vi "DSC Dashboard.vi"() -> ()   [LabVIEW 2016]
uses:
  <vilib>/addons/_JKI.lib/REST Client/classes/REST Client/HTTP Header.ctl
  OAuth/OO OAuth/scope_needed.ctl
  <vilib>/Platform/browser.llb/Open URL in Default Browser (string).vi
  <vilib>/regexp/Match Regular Expression.xnode
  <vilib>/addons/_JKI.lib/REST Client/classes/REST Client/REST Client.lvclass
  <vilib>/addons/_JKI.lib/Serialization/JSON/JKI JSON Serialization.lvlib
panel:
  out "Last Update":string
  in  "Go to Asana":bool
  in  "Add new value":bool
  in  "Update Button":bool
  in  "OK":bool
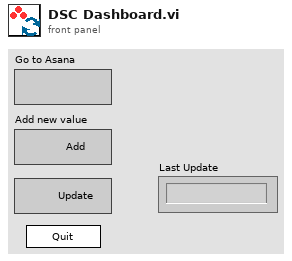
[diagram p1: front panel]
types:
  T1 = enum32{"Invalid", "Standard", "Closed", "Hidden", "Minimized", "Maximized"}
  T2 = enum32{"invalid app kind", "Development System", "Run Time System", "Student Edition", "Embedded LabVIEW", "Evaluation", "Custom"}
  T3 = cluster{"Client ID":string, "Client Secret":string, "Redirect URI":string, "Token Endpoint":string, "Scope":string}
  T4 = typedef "scope_needed.ctl" = enum16{"No", "Yes"}
  T5 = typedef "REST Client.lvlib/REST Client.lvclass/HTTP Header.ctl" = cluster{"header":string, "value":string}
  T6 = cluster{"Core":cluster{"Current VI Reference":refnum<vi>, "Close Panel on Exit?":bool}, "Access Token":string, "Auth Timeout":dbl, "Refresh Token":string, "DSC Data + GID":cluster{dbl, string}[], "headers":T5[]}
  T7 = cluster{"Current VI Reference":refnum<vi>, "Close Panel on Exit?":bool}
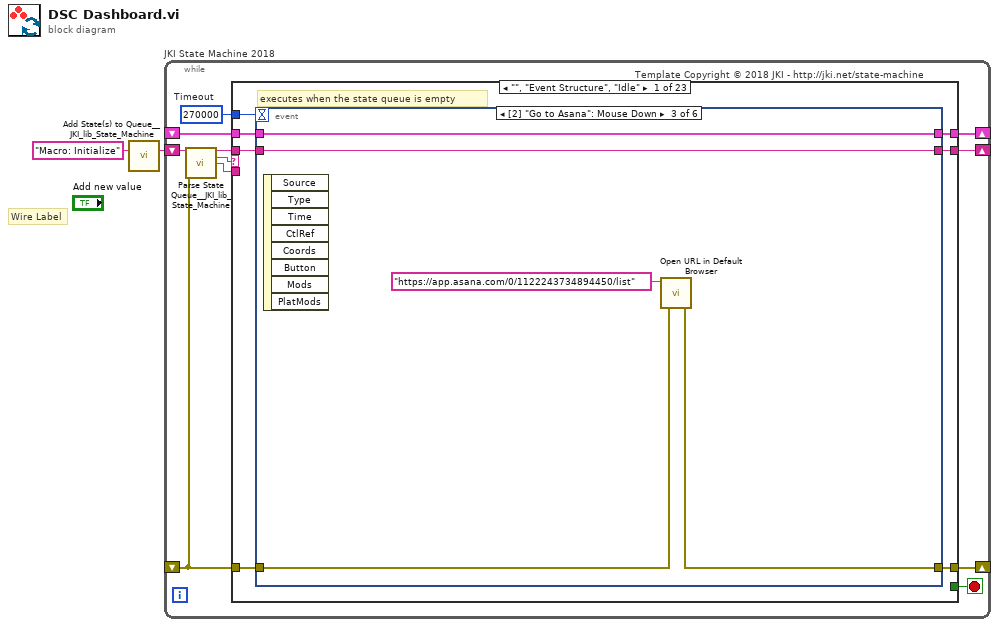
[diagram p0: block diagram]
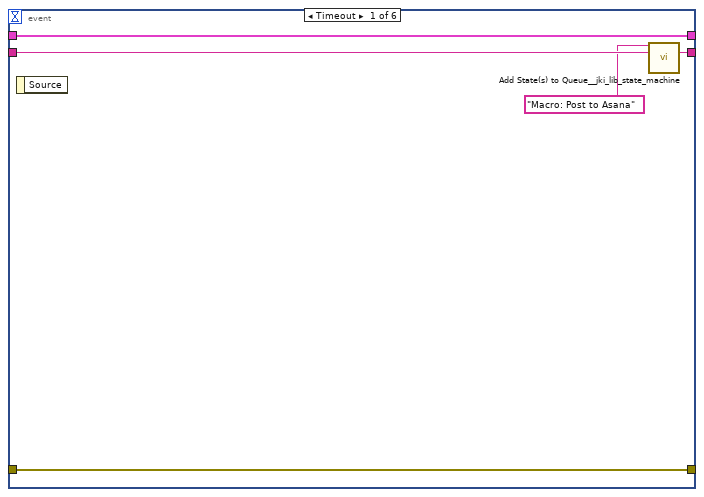
[diagram p2: hidden frame]
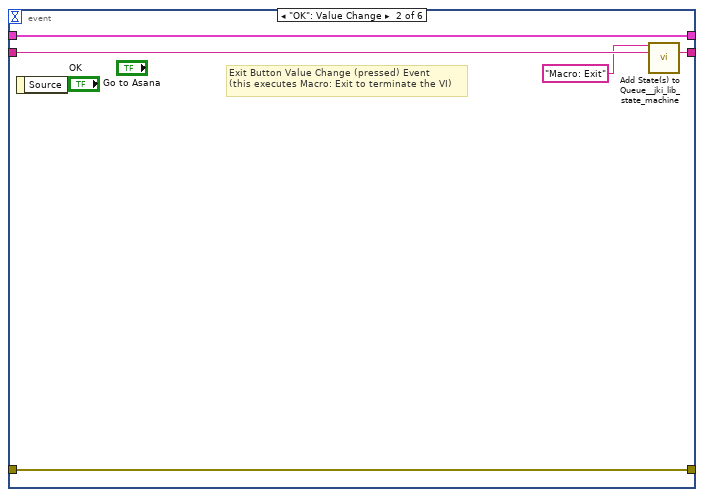
[diagram p3: hidden frame]
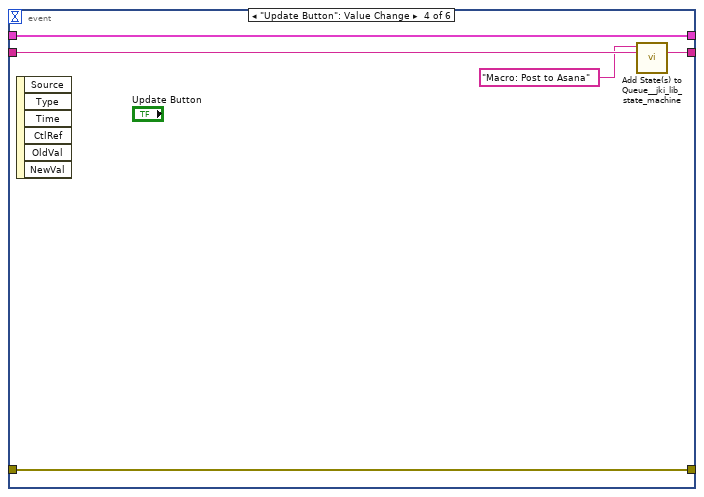
[diagram p4: hidden frame]
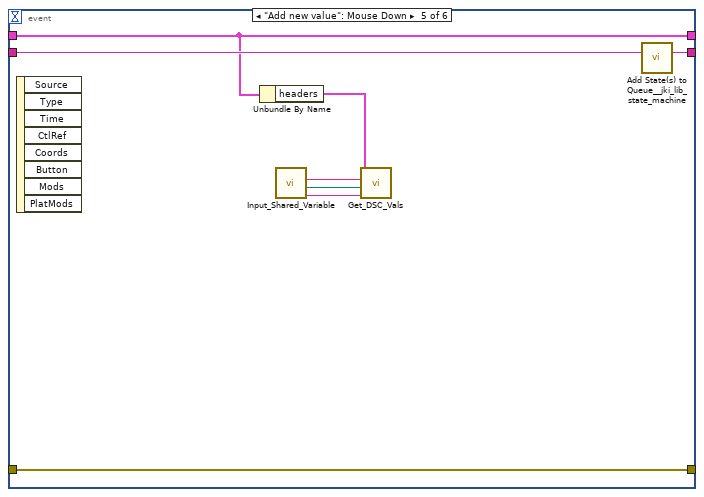
[diagram p5: hidden frame]
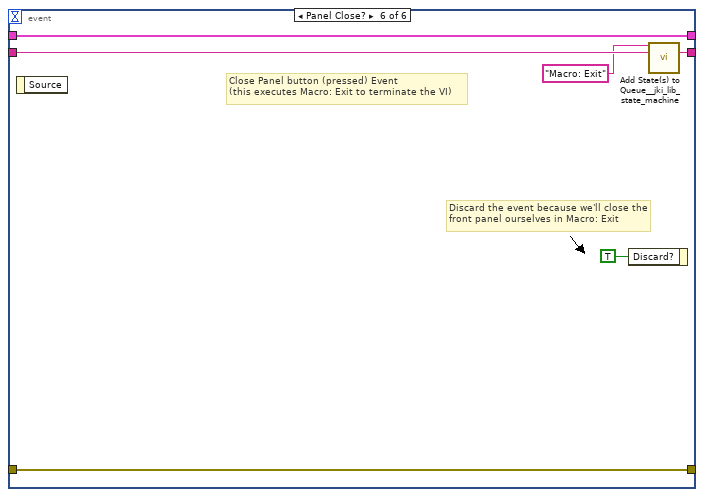
[diagram p6: hidden frame]
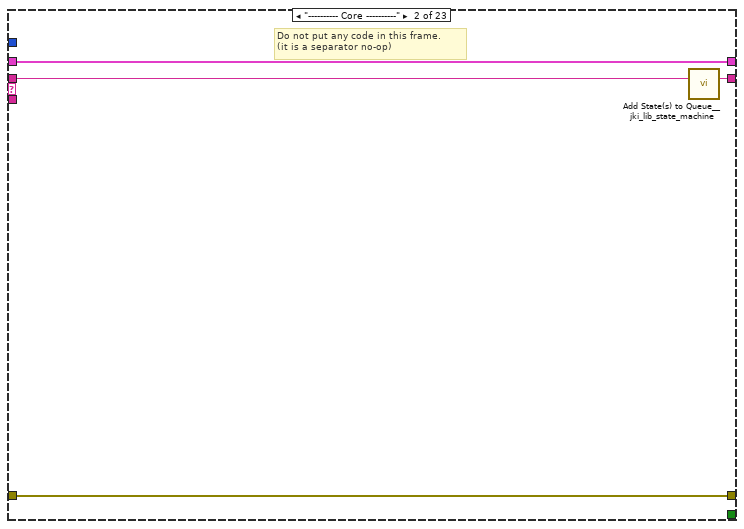
[diagram p7: hidden frame]
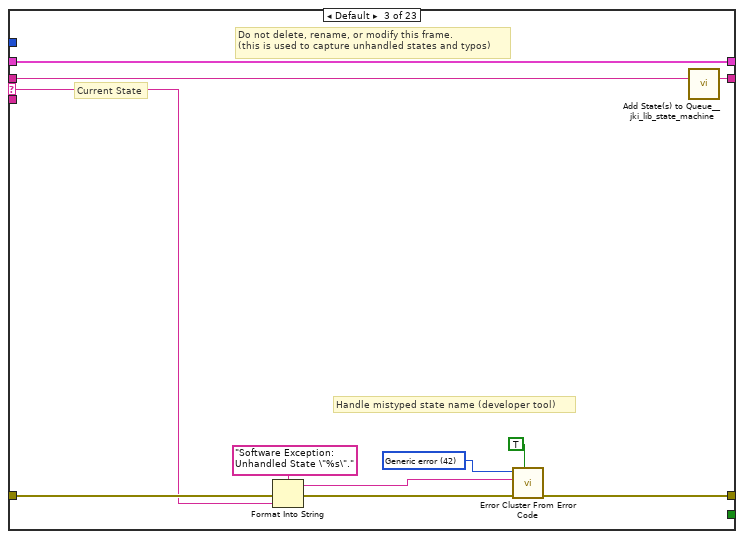
[diagram p8: hidden frame]
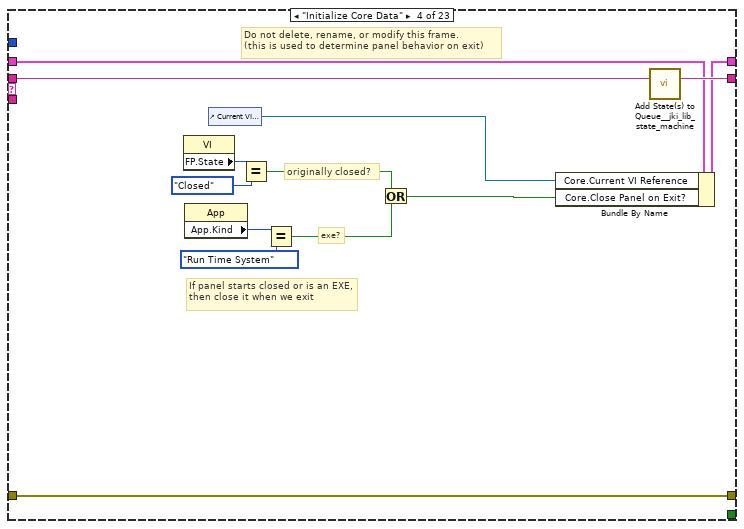
[diagram p9: hidden frame]
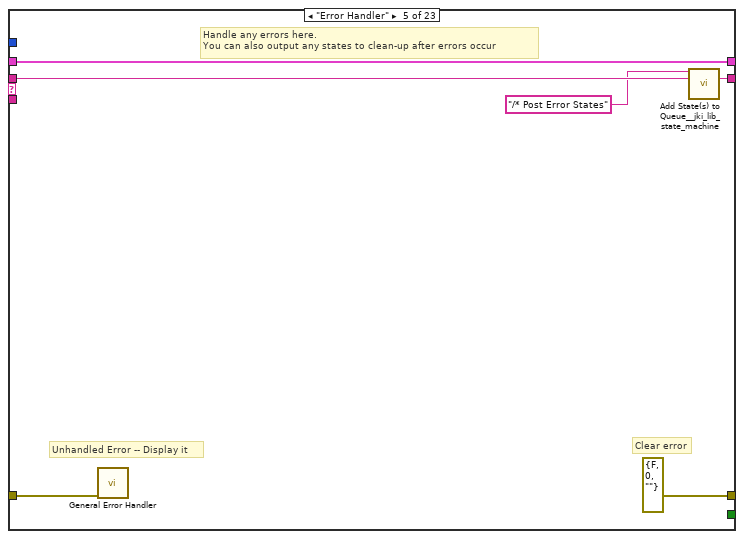
[diagram p10: hidden frame]
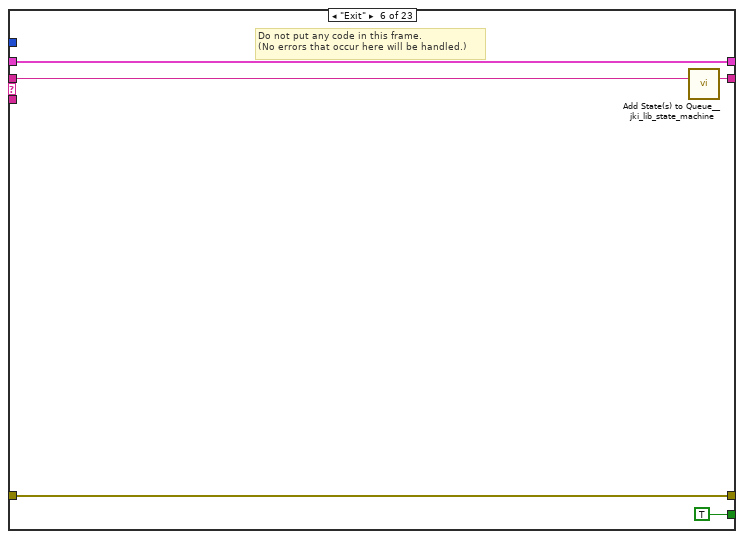
[diagram p11: hidden frame]
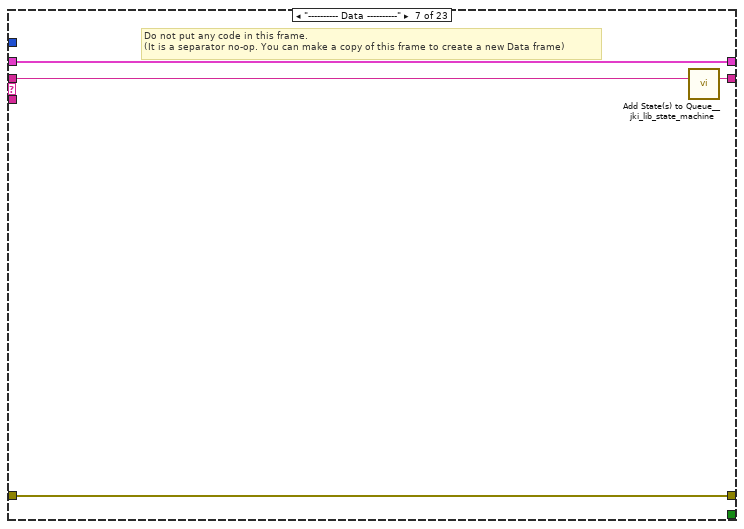
[diagram p12: hidden frame]
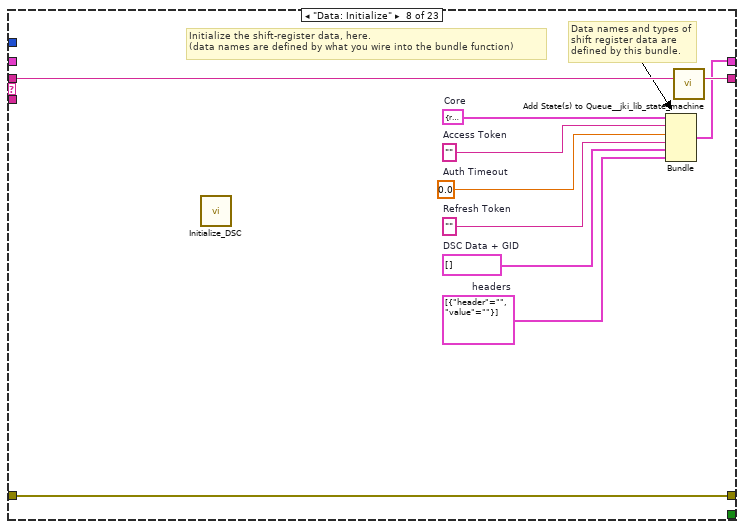
[diagram p13: hidden frame]
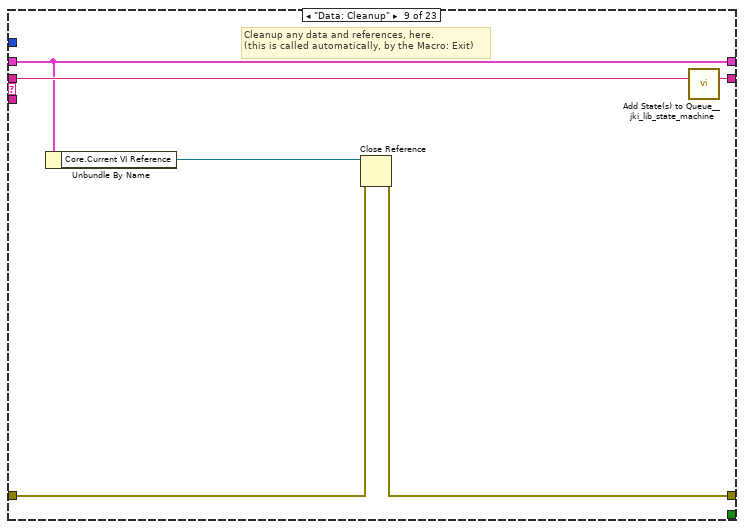
[diagram p14: hidden frame]
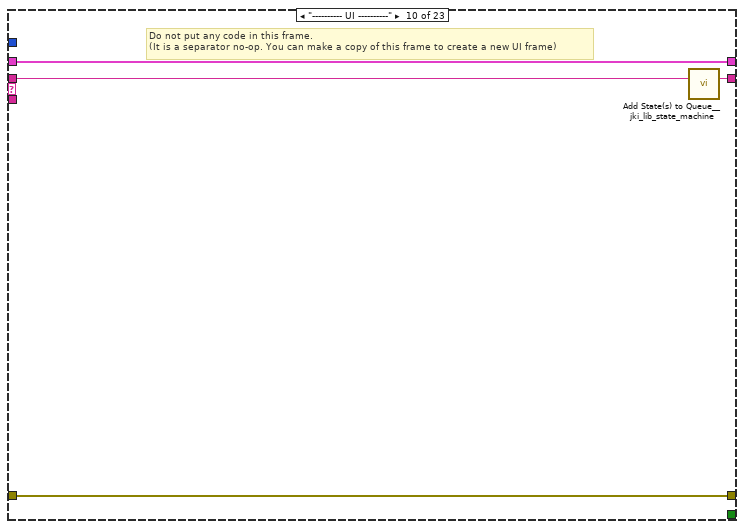
[diagram p15: hidden frame]
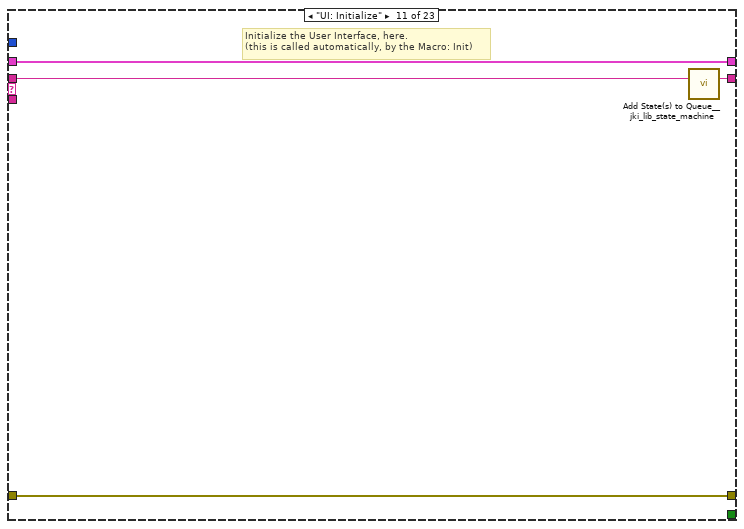
[diagram p16: hidden frame]
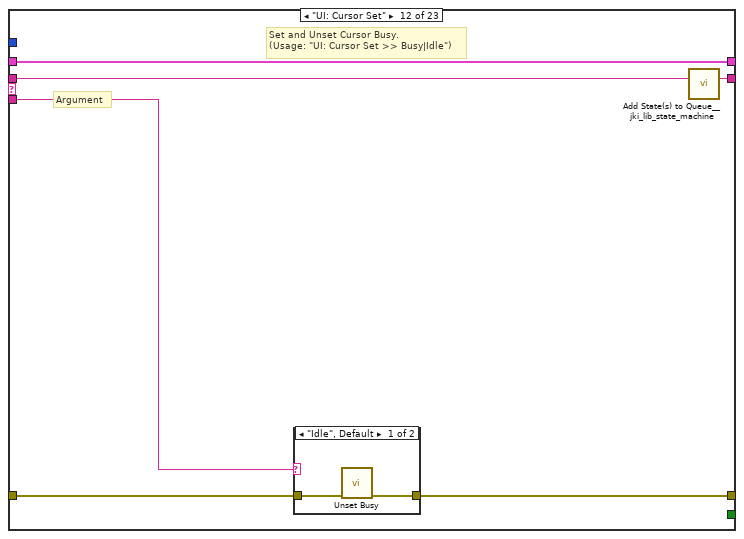
[diagram p17: hidden frame]
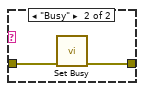
[diagram p18: hidden frame]
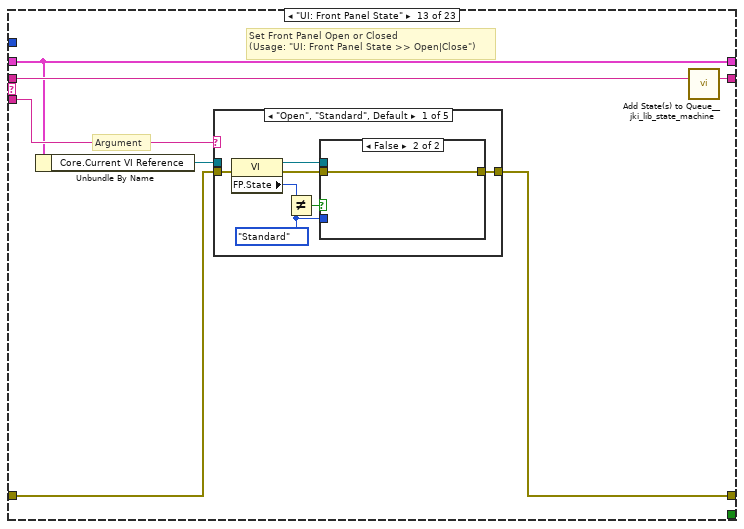
[diagram p19: hidden frame]
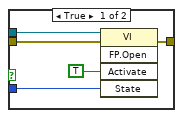
[diagram p20: hidden frame]
diagram:
  # "Wire Label"
  n1 = call <vilib>:"Add State(s) to Queue__JKI_lib_State_Machine.vi"("State(s) in (\"\")"="Macro: Initialize") -> ("States Out"=w2:string)  [unwired: 14 in]
  n2 = while "JKI State Machine 2018" {
    shift-right: [w3] -> _
    shift-left: _ -> [w6]
    shift-right: [w9] -> _
    shift-left: _ -> [w4]
    shift-right: [w8] -> _
    shift-left: w2 -> [w10]
    stop <- w7 stop-if-true
    w5 = 270000  # Timeout
    # "Template Copyright © 2018 JKI - http://jki.net/state-machine"
    n3 = call <vilib>:"Parse State Queue__JKI_lib_State_Machine.vi"("State Queue"=w10, "Error In (no error)"=w4) -> ("Remaining States"=w12:string, "Current State"=w13:string, "Arguments"=w11:string)  [unwired: 11 in]
    n4 = case shown="\"\", \"Event Structure\", \"Idle\"" w13 {
      selector: w13 -> [_ _ w59 _ _ _ _ _ _ _ _ _ _ _ _ _ _ _ _ _ _ _ _]
      tunnel: w12 -> [w20 w58 w63 w82 w88 w93 w97 w107 w113 w117 w121 w127 w138 w202 w207 w212 w222 w226 w237 w253 w269 w287 w297]
      tunnel: w11 -> [_ _ _ _ _ _ _ _ _ _ _ w122 w133 _ _ _ _ _ _ _ _ _ _]
      tunnel: w6 -> [w18 w55 w61 w71 w85 w91 w94 _ w109 w114 w119 w125 w132 w199 w204 w209 w214 w223 w228 w250 w255 w284 w294]
      tunnel: [w17 w56 w65 w80 errorcluster {"status"=FALSE, "code"=0, "source"=""} ("error out") w90 w95 w105 w110 w115 w118 w123 w135 w200 w205 w210 w220 w224 w231 w251 w260 w285 w295] -> w9
      tunnel: w4 -> [w16 w56 w64 w80 w84 w90 w95 w105 w111 w115 w118 w124 w136 w200 w205 w210 w220 w224 w232 w251 w265 w285 w295]
      tunnel: [w19 w57 w62 w81 w87 w92 w96 w106 w112 w116 w120 w126 w137 w201 w206 w211 w221 w225 w236 w252 w268 w286 w296] -> w8
      tunnel: [_ _ _ _ _ TRUE _ _ _ _ _ _ _ _ _ _ _ _ _ _ _ _ _] -> w7
      tunnel: w5 -> [w14 _ _ _ _ _ _ _ _ _ _ _ _ _ _ _ _ _ _ _ _ _ _]
      tunnel: [w15 w55 w61 w70 w85 w91 w94 w98 w109 w114 w119 w125 w132 w199 w204 w209 w214 w223 w227 w250 w254 w284 w294] -> w3
      frame "", "Event Structure", "Idle" {
        # "executes when the state queue is empty"
        n5 = event shown="[2] \"Go to Asana\": Mouse Down" {
          selector: _ -> [_ _ _ _ _ _]
          dyn-events: _ -> [_ _ _ _ _ _]
          timeout: w14 -> [_ _ _ _ _ _]
          tunnel: w20 -> [w25 w30 w34 w38 w47 w54]
          tunnel: [w24 w29 w34 w39 w48 w53] -> w19
          tunnel: w18 -> [w22 w27 w35 w40 w44 w51]
          tunnel: [w23 w28 w31 w36 w46 w52] -> w17
          tunnel: w16 -> [w23 w28 w32 w36 w46 w52]
          tunnel: [w22 w27 w35 w40 w44 w51] -> w15
          event Timeout {
            n6 = event-data() -> ()  [unwired: 1 in, 1 out]
            n7 = call <vilib>:"Add State(s) to Queue__jki_lib_state_machine.vi"("State(s) in Front (\"\")"="Macro: Post to Asana" ("State(s) in Front (\"\")"), "State(s) in (\"\")"=w25) -> ("States Out"=w24:string)  [unwired: 13 in]
          }
          event "OK": Value Change {
            # "Exit Button Value Change (pressed) Event\n(this executes Macro: Exit to terminate the VI)"
            n8 = event-data() -> ()  [unwired: 1 in, 1 out]
            n9 = call <vilib>:"Add State(s) to Queue__jki_lib_state_machine.vi"("State(s) in Front (\"\")"="Macro: Exit", "State(s) in (\"\")"=w30) -> ("States Out"=w29:string)  [unwired: 13 in]
          }
          event "Go to Asana": Mouse Down {
            n10 = event-data() -> ()  [unwired: 1 in, 8 out]
            n11 = call-poly <vilib>:"Open URL in Default Browser.vi"("error in (no error)"=w32, "URL"="https://app.asana.com/0/1122243734894450/list") -> ("error out"=w31:errorcluster)  [unwired: 4 in, 1 out]
          }
          event "Update Button": Value Change {
            n12 = event-data() -> ()  [unwired: 1 in, 6 out]
            n13 = call <vilib>:"Add State(s) to Queue__jki_lib_state_machine.vi"("State(s) in Front (\"\")"="Macro: Post to Asana", "State(s) in (\"\")"=w38) -> ("States Out"=w39:string)  [unwired: 13 in]
          }
          event "Add new value": Mouse Down {
            n14 = event-data() -> ()  [unwired: 1 in, 8 out]
            n15 = Unbundle By Name(w44) -> ("headers"=w45:T5[])
            n16 = call "Input_Shared_Variable.vi"() -> ("Machine Out"=w41:string, "Shared Variable Out"=w42:refnum<k21>, "Type out"=w43:string)  [unwired: 9 in]
            n17 = call "Get_DSC_Vals.vi"("Machine"=w41, "Shared Variable Control"=w42, "Name"=w43, "Authorization Header"=w45) -> ()  [unwired: 8 in]
            n18 = call <vilib>:"Add State(s) to Queue__jki_lib_state_machine.vi"("State(s) in (\"\")"=w47) -> ("States Out"=w48:string)  [unwired: 14 in]
          }
          event Panel Close? {
            # "Discard the event because we'll close the front panel ourselves in Macro: Exit"
            # "Close Panel button (pressed) Event\n(this executes Macro: Exit to terminate the VI)"
            n19 = event-data() -> ()  [unwired: 1 in, 1 out]
            n20 = event-data("Discard?"=TRUE) -> ()  [unwired: 1 in, 1 out]
            n21 = call <vilib>:"Add State(s) to Queue__jki_lib_state_machine.vi"("State(s) in Front (\"\")"="Macro: Exit", "State(s) in (\"\")"=w54) -> ("States Out"=w53:string)  [unwired: 13 in]
          }
        }
      }
      frame "---------- Core ----------" {
        # "Do not put any code in this frame.\n(it is a separator no-op)"
        n22 = call <vilib>:"Add State(s) to Queue__jki_lib_state_machine.vi"("State(s) in (\"\")"=w58) -> ("States Out"=w57:string)  [unwired: 14 in]
      }
      frame Default {
        w68 = 42 items=["No error", "Argument error", "Memory is full", "Out of zone", "End of file", "File already open", "Generic file I/O error", "File not found", "File permission error", "Disk is full", "Duplicate path", "Too many files open", "System feature not enabled", "Resource file not found", "Cannot add resource", "Resource not found", "Image not found", "Image memory error", "Pen does not exist", "Config type invalid", "Config token not found", "Config parse error", "Config memory error", "Bad external code format", "Bad external code offset", "External code not present", "Null window", "Destroy window error", "Null menu", "Print aborted", "Bad print record", "Print driver error", "Windows error during printing", "Memory error during printing", "Print dialog error", "Generic print error", "Invalid device refnum", "Device not found", "Device parameter error", "Device unit error", "Cannot open device", "Device call aborted", "Generic error", "Cancelled by user", "Object ID too low", "Object ID too high", "Object not in heap", "Unknown heap", "Unknown object (invalid DefProc)", "Unknown object (DefProc not in table)", "Message out of range", "Invalid (null) method", "Unknown message", "Manager call not supported", "Bad address", "Network operation in progress", "Network operation timed out", "Connection is busy", "Network attribute not supported", "Network error", "Address in use", "System out of memory", "Connection aborted", "Connection refused", "Not connected", "Already connected", "Connection closed", "Initialization error (interapplication manager)", "Bad occurrence", "Wait on unbound occurrence handler", "Occurrence queue overflow", "Datalog type conflict", "Unused", "Unrecognized type (interapplication manager)", "Memory corrupt", "Failed to make temporary DLL", "Old CIN version", "Drag socket not found", "Failed to load drop-object", "Failed to register OLE object", "Failed to release OLE object", "Format specifier type mismatch", "Unknown format specifier", "Too few format specifiers", "Too many format specifiers", "Scan failed", "Newer CIN version", "Error converting to variant", "Runtime menu error", "Password tampered", "Variant attribute not found", "Incompatible variant data type", "Event data is not available", "Event Store is not present", "Occurrence is not found", "Event Queue is not created", "Event info is not available", "Refnum passed is NULL", "Error retrieving Class GUID", "Error retrieving CoClass GUID", "Error retrieving TypeLib GUID.", "Bad built application magic bytes.", "Specific driver is different from the specific driver associated with the Logical Name.", "There is no session opened to the class driver.", "Max Error", "MAX - Error with config objects", "MAX - Error loading configuration", "MAX - Group not supported"]
        # "Current State"
        # "Do not delete, rename, or modify this frame.\n(this is used to capture unhandled states and typos)"
        # "Handle mistyped state name (developer tool)"
        n23 = Format Into String(format string="Software Exception: Unhandled State \"%s\"." ("message"), error in=w64, w59) -> (resulting string=w67:string, error out=w66:errorcluster)  [unwired: 1 in]
        n24 = call <vilib>:"Error Cluster From Error Code.vi"("show call chain? (False)"=TRUE, "error in (no error)"=w66, "error message (\"\")"=w67, "error code (0)"=w68) -> ("error out"=w65:errorcluster)  [unwired: 5 in]
        n25 = call <vilib>:"Add State(s) to Queue__jki_lib_state_machine.vi"("State(s) in (\"\")"=w63) -> ("States Out"=w62:string)  [unwired: 14 in]
      }
      frame "Initialize Core Data" {
        # "Do not delete, rename, or modify this frame.\n(this is used to determine panel behavior on exit)"
        # "originally closed?"
        # "exe?"
        # "If panel starts closed or is an EXE, then close it when we exit"
        n26 = property class="VI"() -> ("FP.State"=w74:T1)  [unwired: 2 in, 2 out]
        n27 = property class="App"() -> ("App.Kind"=w79:T2)  [unwired: 2 in, 2 out]
        n28 = control-ref of="Current VI Reference"() -> (w75:refnum<vi>)
        n29 = Equal?(x=w74, y=T1."Closed" ("Front Panel Window:State")) -> (x = y?=w72:bool)
        n30 = Equal?(x=w79, y=T2."Run Time System" ("Application:Kind")) -> (x = y?=w77:bool)
        n31 = Or(x=w72, y=w77) -> (x .or. y?=w76:bool)
        n32 = Bundle By Name(cluster=w71, "Core.Current VI Reference"=w75, "Core.Close Panel on Exit?"=w76) -> (w70:T6)
        n33 = call <vilib>:"Add State(s) to Queue__jki_lib_state_machine.vi"("State(s) in (\"\")"=w82) -> ("States Out"=w81:string)  [unwired: 14 in]
      }
      frame "Error Handler" {
        # "Unhandled Error -- Display it"
        # "Handle any errors here.\nYou can also output any states to clean-up after errors occur"
        # "Clear error"
        n34 = call <vilib>:"General Error Handler.vi"("error in (no error)"=w84) -> ()  [unwired: 10 in, 5 out]
        n35 = call <vilib>:"Add State(s) to Queue__jki_lib_state_machine.vi"("State(s) in Front (\"\")"="/* Post Error States", "State(s) in (\"\")"=w88) -> ("States Out"=w87:string)  [unwired: 13 in]
      }
      frame "Exit" {
        # "Do not put any code in this frame.\n(No errors that occur here will be handled.)"
        n36 = call <vilib>:"Add State(s) to Queue__jki_lib_state_machine.vi"("State(s) in (\"\")"=w93) -> ("States Out"=w92:string)  [unwired: 14 in]
      }
      frame "---------- Data ----------" {
        # "Do not put any code in this frame.\n(It is a separator no-op. You can make a copy of this frame to create a new Data frame)"
        n37 = call <vilib>:"Add State(s) to Queue__jki_lib_state_machine.vi"("State(s) in (\"\")"=w97) -> ("States Out"=w96:string)  [unwired: 14 in]
      }
      frame "Data: Initialize" {
        w99 = cluster{dbl, string}[] []  # DSC Data + GID
        w100 = T5[] [{"header"="", "value"=""}]  # headers
        w101 = ""  # Refresh Token
        w102 = ""  # Access Token
        w103 = 0.0  # Auth Timeout
        w104 = T7 {"Current VI Reference"=refnum, "Close Panel on Exit?"=FALSE}  # Core
        # "Data names and types of shift register data are defined by this bundle."
        # "Initialize the shift-register data, here.\n(data names are defined by what you wire into the bundle function)"
        n38 = call "Initialize_DSC.vi"() -> ()  [unwired: 12 in]
        n39 = Bundle("Core"=w104, "Access Token"=w102, "Auth Timeout"=w103, "Refresh Token"=w101, "DSC Data + GID"=w99, "headers"=w100) -> (w98:T6)  [unwired: 1 in]
        n40 = call <vilib>:"Add State(s) to Queue__jki_lib_state_machine.vi"("State(s) in (\"\")"=w107) -> ("States Out"=w106:string)  [unwired: 14 in]
      }
      frame "Data: Cleanup" {
        # "Cleanup any data and references, here.\n(this is called automatically, by the Macro: Exit)"
        n41 = Unbundle By Name(w109) -> ("Core.Current VI Reference"=w108:refnum<vi>)
        n42 = Close Reference(reference=w108, error in (no error)=w111) -> (error out=w110:errorcluster)
        n43 = call <vilib>:"Add State(s) to Queue__jki_lib_state_machine.vi"("State(s) in (\"\")"=w113) -> ("States Out"=w112:string)  [unwired: 14 in]
      }
      frame "---------- UI ----------" {
        # "Do not put any code in this frame.\n(It is a separator no-op. You can make a copy of this frame to create a new UI frame)"
        n44 = call <vilib>:"Add State(s) to Queue__jki_lib_state_machine.vi"("State(s) in (\"\")"=w117) -> ("States Out"=w116:string)  [unwired: 14 in]
      }
      frame "UI: Initialize" {
        # "Initialize the User Interface, here.\n(this is called automatically, by the Macro: Init)"
        n45 = call <vilib>:"Add State(s) to Queue__jki_lib_state_machine.vi"("State(s) in (\"\")"=w121) -> ("States Out"=w120:string)  [unwired: 14 in]
      }
      frame "UI: Cursor Set" {
        # "Argument"
        # "Set and Unset Cursor Busy.\n(Usage: \"UI: Cursor Set >> Busy|Idle\")"
        n46 = case shown="\"Idle\", Default" w122 {
          tunnel: w124 -> [w129 w131]
          tunnel: [w128 w130] -> w123
          frame "Idle", Default {
            n47 = call <vilib>:"Unset Busy.vi"("error in (no error)"=w129) -> ("error out"=w128:errorcluster)  [unwired: 10 in]
          }
          frame "Busy" {
            n48 = call <vilib>:"Set Busy.vi"("error in (no error)"=w131) -> ("error out"=w130:errorcluster)  [unwired: 9 in, 1 out]
          }
        }
        n49 = call <vilib>:"Add State(s) to Queue__jki_lib_state_machine.vi"("State(s) in (\"\")"=w127) -> ("States Out"=w126:string)  [unwired: 14 in]
      }
      frame "UI: Front Panel State" {
        # "Argument"
        # "Set Front Panel Open or Closed\n(Usage: \"UI: Front Panel State >> Open|Close\")"
        n50 = Unbundle By Name(w132) -> ("Core.Current VI Reference"=w134:refnum<vi>)
        n51 = case shown="\"Open\", \"Standard\", Default" w133 {
          tunnel: w136 -> [w144 w157 w168 w180 w192]
          tunnel: [w145 w158 w169 w181 w193] -> w135
          tunnel: w134 -> [_ _ _ _ _]
          frame "Open", "Standard", Default {
            w139 = T1."Standard" ("State")
            n52 = property class="VI"(error in=w144) -> (reference out=w142:refnum<vi>, error out=w143:errorcluster, "FP.State"=w141:T1)  [unwired: 1 in]
            n53 = Not Equal?(x=w141, y=w139) -> (x != y?=w140:bool)
            n54 = case shown="False" w140 {
              tunnel: [w149 w151] -> w145
              tunnel: w143 -> [w148 w151]
              tunnel: w142 -> [w147 _]
              tunnel: w139 -> [w146 _]
              frame True {
                n55 = invoke class="VI" method="FP.Open"(reference=w147, error in=w148, "Activate"=TRUE, "State"=w146) -> (error out=w149:errorcluster)  [unwired: 1 in, 4 out]
              }
              frame False {
              }
            }
          }
          frame "Close", "Closed" {
            n56 = property class="VI"(error in=w157) -> (reference out=w155:refnum<vi>, error out=w156:errorcluster, "FP.State"=w153:T1)  [unwired: 1 in]
            n57 = Not Equal?(x=w153, y=T1."Closed" ("Front Panel Window:State")) -> (x != y?=w152:bool)
            n58 = case shown="True" w152 {
              tunnel: [w159 w162] -> w158
              tunnel: w156 -> [w159 w161]
              tunnel: w155 -> [_ w160]
              frame False {
              }
              frame True {
                n59 = invoke class="VI" method="FP.Close"(reference=w160, error in=w161) -> (error out=w162:errorcluster)  [unwired: 1 in, 2 out]
              }
            }
          }
          frame "Hidden", "Hide" {
            w163 = T1."Hidden" ("State")
            n60 = property class="VI"(error in=w168) -> (reference out=w166:refnum<vi>, error out=w167:errorcluster, "FP.State"=w165:T1)  [unwired: 1 in]
            n61 = Not Equal?(x=w165, y=w163) -> (x != y?=w164:bool)
            n62 = case shown="True" w164 {
              tunnel: [w173 w174] -> w169
              tunnel: w167 -> [w172 w174]
              tunnel: w166 -> [w171 _]
              tunnel: w163 -> [w170 _]
              frame True {
                n63 = invoke class="VI" method="FP.Open"(reference=w171, error in=w172, "State"=w170) -> (error out=w173:errorcluster)  [unwired: 2 in, 4 out]
              }
              frame False {
              }
            }
          }
          frame "Minimize", "Minimized" {
            w175 = T1."Minimized" ("State")
            n64 = property class="VI"(error in=w180) -> (reference out=w178:refnum<vi>, error out=w179:errorcluster, "FP.State"=w177:T1)  [unwired: 1 in]
            n65 = Not Equal?(x=w177, y=w175) -> (x != y?=w176:bool)
            n66 = case shown="True" w176 {
              tunnel: [w185 w186] -> w181
              tunnel: w179 -> [w184 w186]
              tunnel: w178 -> [w183 _]
              tunnel: w175 -> [w182 _]
              frame True {
                n67 = invoke class="VI" method="FP.Open"(reference=w183, error in=w184, "State"=w182) -> (error out=w185:errorcluster)  [unwired: 2 in, 4 out]
              }
              frame False {
              }
            }
          }
          frame "Maximize", "Maximized" {
            w187 = T1."Maximized" ("State")
            n68 = property class="VI"(error in=w192) -> (reference out=w190:refnum<vi>, error out=w191:errorcluster, "FP.State"=w189:T1)  [unwired: 1 in]
            n69 = Not Equal?(x=w189, y=w187) -> (x != y?=w188:bool)
            n70 = case shown="True" w188 {
              tunnel: [w197 w198] -> w193
              tunnel: w191 -> [w196 w198]
              tunnel: w190 -> [w195 _]
              tunnel: w187 -> [w194 _]
              frame True {
                n71 = invoke class="VI" method="FP.Open"(reference=w195, error in=w196, "State"=w194) -> (error out=w197:errorcluster)  [unwired: 2 in, 4 out]
              }
              frame False {
              }
            }
          }
        }
        n72 = call <vilib>:"Add State(s) to Queue__jki_lib_state_machine.vi"("State(s) in (\"\")"=w138) -> ("States Out"=w137:string)  [unwired: 14 in]
      }
      frame "---------- Macro ----------" {
        # "Do not put any code in this frame.\n(It is a separator no-op. You can make a copy of this frame to create a new Macro frame)"
        n73 = call <vilib>:"Add State(s) to Queue__jki_lib_state_machine.vi"("State(s) in (\"\")"=w202) -> ("States Out"=w201:string)  [unwired: 14 in]
      }
      frame "Macro: Post to Asana" {
        # "Do not put any code in this frame.\n(It is a separator no-op. You can make a copy of this frame to create a new Macro frame)"
        n74 = call <vilib>:"Add State(s) to Queue__jki_lib_state_machine.vi"("State(s) in Front (\"\")"="Authorization: Handle\nDSC: Get DSC Values\nAsana: Post Values" ("State(s) in Front (\"\")"), "State(s) in (\"\")"=w207) -> ("States Out"=w206:string)  [unwired: 13 in]
      }
      frame "Macro: Initialize" {
        w208 = "Data: Initialize\nInitialize Core Data\nUI: Initialize\nUI: Front Panel State >> Open\nMacro: Post to Asana"  # Data: Initialize Initialize Core Data UI: Initialize UI: Front Panel State >> Open Macro: Post to Asana
        # "Initialization Macro\n(This is called once, when the VI starts)"
        n75 = call <vilib>:"Add State(s) to Queue__jki_lib_state_machine.vi"("State(s) in Front (\"\")"=w208, "State(s) in (\"\")"=w212) -> ("States Out"=w211:string)  [unwired: 13 in]
      }
      frame "Macro: Exit" {
        # "Exit Macro\n(This is called once, when the VI exits)"
        n76 = Unbundle By Name(w214) -> ("Core.Close Panel on Exit?"=w213:bool)
        n77 = Select(t="UI: Front Panel State >> Close", s=w213, f="") -> (s? t:f=w217:string)
        n78 = call <vilib>:"Add State(s) to Queue__jki_lib_state_machine.vi"("State(s) in (\"\")"=w217, "State(s) at Back (\"\")"="Data: Cleanup\nExit") -> ("States Out"=w215:string)  [unwired: 13 in]
        n79 = call <vilib>:"Add State(s) to Queue__jki_lib_state_machine.vi"("State(s) in Front (\"\")"=w215, "State(s) in (\"\")"=w222) -> ("States Out"=w221:string)  [unwired: 13 in]
      }
      frame "---------- Authorization ----------" {
        # "Template Separator\n(You can make a copy of, or modify, this frame)"
        n80 = call <vilib>:"Add State(s) to Queue__jki_lib_state_machine.vi"("State(s) in (\"\")"=w226) -> ("States Out"=w225:string)  [unwired: 14 in]
      }
      frame "Authorization: Handle" {
        # "If it is, reauthenticate.\nIf not, do nothing."
        # "Check if the current time is\ngreater than the authentication\ndeadline"
        n81 = Get Date/Time In Seconds() -> (seconds since 1Jan1904=w235:timestamp)
        n82 = Unbundle By Name(w228) -> ("Auth Timeout"=w229:dbl, "Refresh Token"=w230:string)
        n83 = To Double Precision Float(number=w235) -> (double precision float=w233:dbl)
        n84 = Less Or Equal?(x=w229, y=w233) -> (x <= y?=w234:bool)
        n85 = case shown="True" w234 {
          tunnel: w232 -> [w239 w248]
          tunnel: [w239 w247] -> w231
          tunnel: [w238 w246] -> w227
          tunnel: w230 -> [_ _]
          tunnel: w228 -> [w238 w242]
          frame False {
          }
          frame True {
            n86 = call "Authenticate.vi"("error in (no error)"=w248, "Authentication Info"=T3 {"Client ID"="1108428692000476", "Client Secret"="803bdca1138fccb00921b8f346728904", "Redirect URI"="https://app.asana.com/api/1.0", "Token Endpoint"="https://app.asana.com/-/oauth_token", "Scope"=""}, "Scope Needed?"=scope_needed."No") -> ("error out"=w247:errorcluster, "Refresh Token"=w243:string, "Timeout"=w249:dbl, "Access Token"=w240:string)  [unwired: 5 in]
            n87 = call "Authentication_Header_Handler.vi"("String"=w240) -> ("output array"=w241:T5[])  [unwired: 10 in]
            n88 = Bundle By Name(cluster=w242, "headers"=w241, "Auth Timeout"=w249, "Refresh Token"=w243) -> (w246:T6)
          }
        }
        n89 = call <vilib>:"Add State(s) to Queue__jki_lib_state_machine.vi"("State(s) in (\"\")"=w237) -> ("States Out"=w236:string)  [unwired: 14 in]
      }
      frame "---------- DSC ----------" {
        # "Template Separator\n(You can make a copy of, or modify, this frame)"
        n90 = call <vilib>:"Add State(s) to Queue__jki_lib_state_machine.vi"("State(s) in (\"\")"=w253) -> ("States Out"=w252:string)  [unwired: 14 in]
      }
      frame "DSC: Get DSC Values" {
        w258 = cluster{string, string}[] []
        n91 = call <vilib>:"Application Directory.vi"() -> ("Application Directory"=w264:path)
        n92 = Build Path(base path=w264, name or relative path="DSC_Variables.json") -> (appended path=w267:path)
        n93 = Read from Text File(file (use dialog)=w267, error in=w265) -> (text=w259:string, error out=w262:errorcluster)  [unwired: 2 in, 2 out]
        n94 = call <vilib>:"Unflatten From JSON String.vi"("Type and Defaults"=w258, "error in (no error)"=w262, "JSON String"=w259) -> ("error out"=w261:errorcluster, "Variant"=w263:variant)  [unwired: 7 in]
        n95 = Variant To Data(error in=w261, type=w258, Variant=w263) -> (data=w256:cluster{string, string}[], error out=w260:errorcluster)
        n96 = for {
          tunnel: [w278] -> w257 mode=indexing
          tunnel: w256 -> [w276] mode=indexing
          n97 = Unbundle(w276) -> (w275:string, w274:string)
          n98 = Variant To Data(type=refnum<k21> refnum ("shared variable refnum in"), Variant=w275) -> (data=w282:refnum<k21>)  [unwired: 1 in, 1 out]
          n99 = shared-variable-open(w282, 0.0) -> (w281:refnum<k21>, w273:errorcluster)  [unwired: 2 in]
          n100 = shared-variable-read(w281) -> (w280:refnum<k21>, w272:errorcluster, w279:dbl)  [unwired: 1 in, 1 out]
          n101 = call <vilib>:"Clear Errors.vi"("error in (no error)"=w273, "specific error code to clear (0: all)"=0) -> ()  [unwired: 4 in, 2 out]
          n102 = Close Variable Connection(11:w280) -> ()  [unwired: 1 in, 1 out]
          n103 = call <vilib>:"Clear Errors.vi"("error in (no error)"=w272, "specific error code to clear (0: all)"=0) -> ()  [unwired: 4 in, 2 out]
          n104 = Bundle(w279, w274) -> (w278:cluster{dbl, string})  [unwired: 1 in]
        }
        n105 = Bundle By Name(cluster=w255, "DSC Data + GID"=w257) -> (w254:T6)
        n106 = call <vilib>:"Add State(s) to Queue__jki_lib_state_machine.vi"("State(s) in (\"\")"=w269) -> ("States Out"=w268:string)  [unwired: 14 in]
      }
      frame "---------- Asana ----------" {
        # "Template Separator\n(You can make a copy of, or modify, this frame)"
        n107 = call <vilib>:"Add State(s) to Queue__jki_lib_state_machine.vi"("State(s) in (\"\")"=w287) -> ("States Out"=w286:string)  [unwired: 14 in]
      }
      frame "Asana: Post Values" {
        n108 = Unbundle By Name(w294) -> ("DSC Data + GID"=w293:cluster{dbl, string}[], "headers"=w292:T5[])
        n109 = call <vilib>:"Create REST Client.vi"("Base URL"="https://app.asana.com/api/1.0") -> ("REST Client out"=w290:refnum<class "REST Client.lvclass">)  [unwired: 9 in, 1 out]
        n110 = for {
          tunnel: w293 -> [w313] mode=indexing
          tunnel: w292 -> [w306]
          tunnel: w290 -> [w305]
          tunnel: [w310] -> w289
          n111 = Unbundle(w313) -> (w311:dbl, w312:string)
          n112 = Format Into String(w311) -> (resulting string=w308:string)  [unwired: 3 in, 1 out]
          n113 = Concatenate Strings("/tasks/" ("string"), w312) -> (w307:string)
          n114 = call <vilib>:"Application Directory.vi"() -> ("Application Directory"=w301:path)
          n115 = call-dynamic "HTTP GET.vi"("request specific headers"=w306, "Path"=w307, "REST Client in"=w305) -> ("Response body"=w302:string, "REST Client out"=w309:refnum<class "REST Client.lvclass">)  [unwired: 3 in, 4 out]
          n116 = Build Path(base path=w301, name or relative path="Task_Name_Search.txt") -> (appended path=w300:path)
          n117 = Read from Text File(file (use dialog)=w300) -> (text=w299:string)  [unwired: 3 in, 3 out]
          n118 = xnode "Match Regular Expression"("input string"=w302, "regular expression"=w299) -> ("whole match"=w303:string)  [unwired: 4 in, 4 out]
          n119 = Concatenate Strings("{\"data\": {\"name\": \"" ("Request body"), w303, w308, "\"}}" ("string")) -> (w314:string)
          n120 = call-dynamic "HTTP PUT.vi"("request specific headers"=w306, "Request body"=w314, "Path"=w307, "REST Client in"=w309) -> ("REST Client out"=w310:refnum<class "REST Client.lvclass">)  [unwired: 2 in, 5 out]
        }
        n121 = Get Date/Time String() -> (time string=→"Last Update":string)  [unwired: 3 in, 1 out]
        n122 = call-dynamic "Destroy REST Client.vi"("REST Client in"=w289) -> ()  [unwired: 10 in, 1 out]
        n123 = call <vilib>:"Add State(s) to Queue__jki_lib_state_machine.vi"("State(s) in (\"\")"=w297) -> ("States Out"=w296:string)  [unwired: 14 in]
      }
    }
  }
